vi "PLC Unpuck.vi"(7 "PVT in":T1={"Mode"=1, "Pressure PV"=0.0, "Pressure SP"=0.0, "Flow PV"=0.0, "Flow SP"=0.0, "Volume PV"=0.0, "Volume SP"=0.0, "MM PV"=0.0, "Start"=FALSE, "Home"=FALSE} {"Mode" items=["Pressure"=1, "Flow"=2, "Volume"=3]}, 11 "register values":u16[](array[numeric])) -> (3 "PVT":T1={"Mode"=1, "Pressure PV"=0.0, "Pressure SP"=0.0, "Flow PV"=0.0, "Flow SP"=0.0, "Volume PV"=0.0, "Volume SP"=0.0, "MM PV"=0.0, "Start"=FALSE, "Home"=FALSE} {"Mode" items=["Pressure"=1, "Flow"=2, "Volume"=3]})   [LabVIEW 2023, in "Drive.lvlib"]
uses:
  Drive.lvlib
  PVT_Drive_Type.ctl
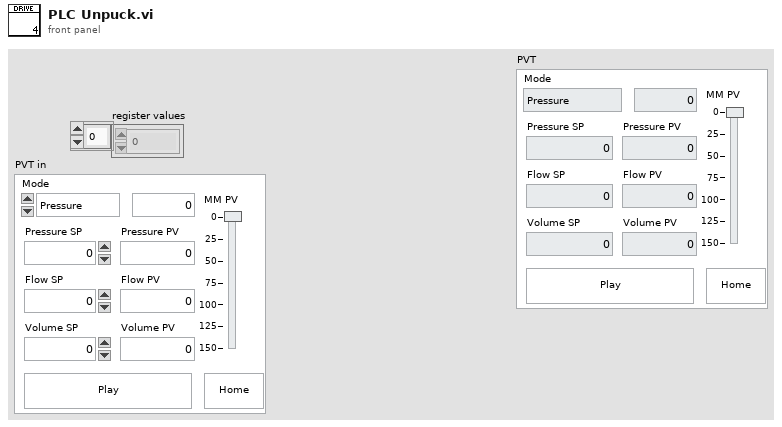
[diagram p1: front panel]
types:
  T1 = typedef "Drive.lvlib/PVT_Drive_Type.ctl" = cluster{"Mode":u16, "Pressure PV":dbl, "Pressure SP":dbl, "Flow PV":dbl, "Flow SP":dbl, "Volume PV":dbl, "Volume SP":dbl, "MM PV":dbl, "Start":bool, "Home":bool}
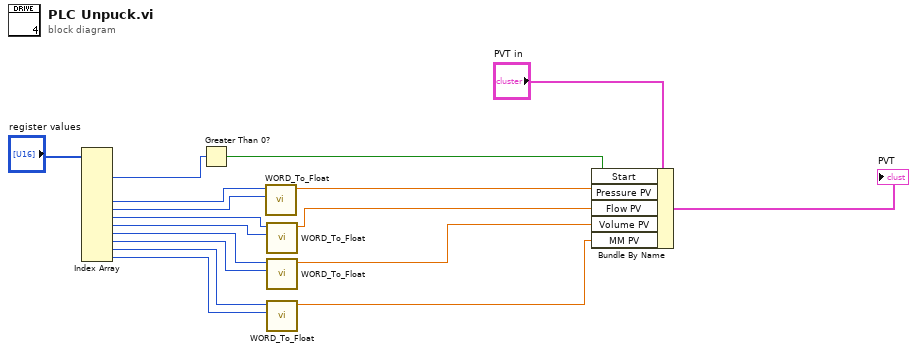
[diagram p0: block diagram]
diagram:
  n1 = Index Array(array="register values") -> (element #2=w16:u16, element #5=w12:u16, element #6=w11:u16, element #7=w10:u16, element #8=w9:u16, element #9=w8:u16, element #10=w7:u16, element #11=w3:u16, element #12=w2:u16)  [unwired: 12 in, 3 out]
  n2 = Greater Than 0?(x=w16) -> (x > 0?=w14:bool)
  n3 = call "WORD_To_Float.vi"("second_Word"=w11, "first_Word"=w12) -> ("output_Float"=w6:sgl)  [unwired: 9 in]
  n4 = call "WORD_To_Float.vi"("second_Word"=w9, "first_Word"=w10) -> ("output_Float"=w5:sgl)  [unwired: 9 in]
  n5 = call "WORD_To_Float.vi"("second_Word"=w7, "first_Word"=w8) -> ("output_Float"=w4:sgl)  [unwired: 9 in]
  n6 = call "WORD_To_Float.vi"("second_Word"=w2, "first_Word"=w3) -> ("output_Float"=w1:sgl)  [unwired: 9 in]
  n7 = Bundle By Name(cluster="PVT in", "Start"=w14, "Pressure PV"=w6, "Flow PV"=w5, "Volume PV"=w4, "MM PV"=w1) -> (→"PVT":T1)
